vi "generateSweep.vi"(0 "Sweep type":u16(ring) items=["Linear", "Logarithmic"], 5 "Points or Points/Decade":u16=10 min=1 step=1, 7 "Start frequency":dbl=1000.0 min=0.0 step=1000.0 format="%.2p", 9 "Stop frequency":dbl=10000.0 min=0.0 step=1000.0 format="%.2p", 11 "error in (no error)":errorcluster) -> (4 "Sweep values":dbl[](array[numeric]) format="%_6g", 6 "Count":u32, 15 "error out":errorcluster)   [LabVIEW 2020]
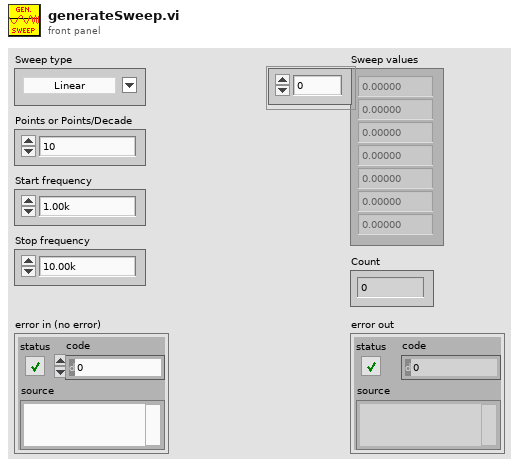
[diagram p1: front panel]
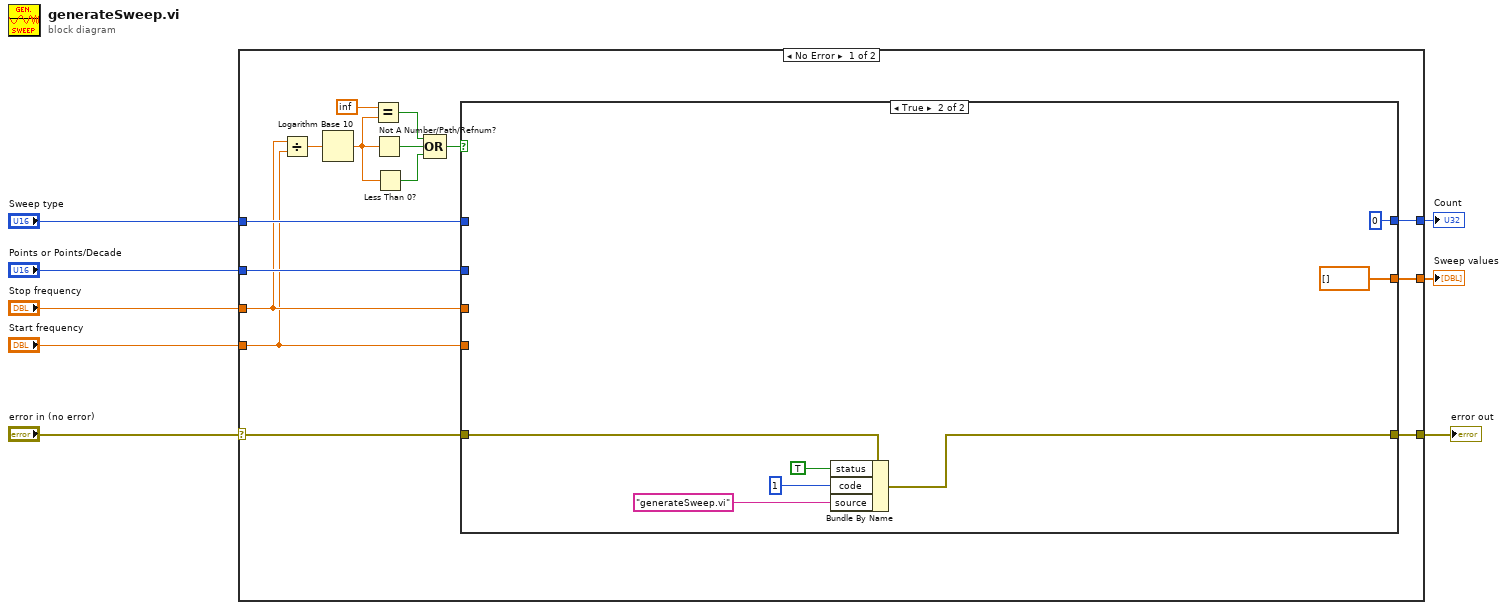
[diagram p0: block diagram]
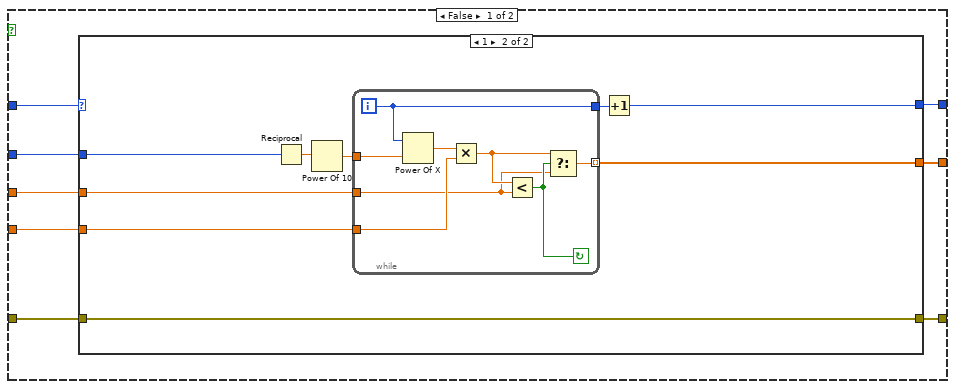
[diagram p2: hidden frame]
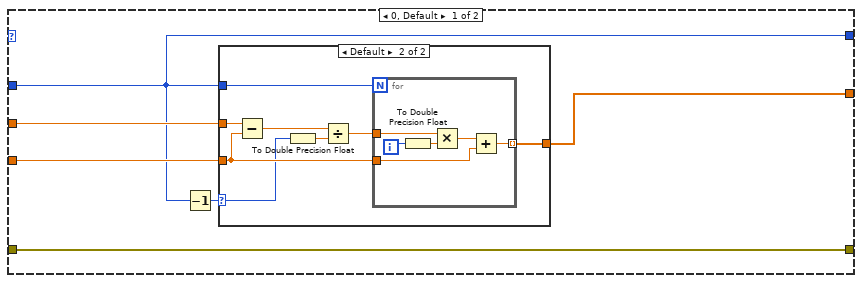
[diagram p3: hidden frame]
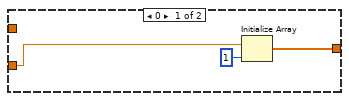
[diagram p4: hidden frame]
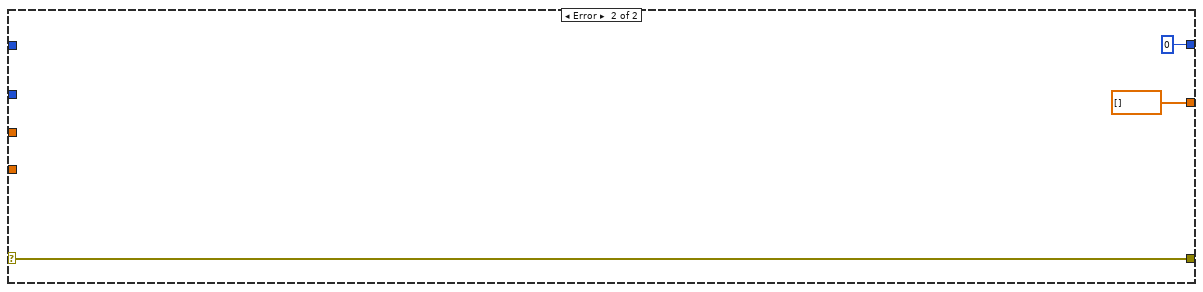
[diagram p5: hidden frame]
diagram:
  n1 = case shown="No Error" "error in (no error)" {
    selector: "error in (no error)" -> [w21 w81]
    tunnel: "Sweep type" -> [w23 _]
    tunnel: "Points or Points/Decade" -> [w22 _]
    tunnel: "Stop frequency" -> [w12 _]
    tunnel: "Start frequency" -> [w11 _]
    tunnel: [w20 w81] -> w3
    tunnel: [w10 0 ("Points or Points/Decade")] -> w2
    tunnel: [w9 dbl[] []] -> w1
    frame No Error {
      n2 = Divide(x=w12, y=w11) -> (x/y=w19:dbl)
      n3 = Logarithm Base 10(1:w19) -> (0:w14:dbl)
      n4 = Equal?(x=inf, y=w14) -> (x = y?=w18:bool)
      n5 = Not A Number/Path/Refnum?(number/path/refnum=w14) -> (NaN/Path/Refnum?=w17:bool)
      n6 = Less Than 0?(x=w14) -> (x < 0?=w16:bool)
      n7 = Compound Arithmetic op=OR(w18, w17, w16) -> (w13:bool)
      n8 = case shown="True" w13 {
        tunnel: w23 -> [w31 _]
        tunnel: w22 -> [w30 _]
        tunnel: w12 -> [w29 _]
        tunnel: w11 -> [w28 _]
        tunnel: w21 -> [w27 w75]
        tunnel: [w26 w74] -> w20
        tunnel: [w25 0 ("Points or Points/Decade")] -> w10
        tunnel: [w24 dbl[] []] -> w9
        frame False {
          n9 = case shown="1" w31 {
            tunnel: w30 -> [w32 w59]
            tunnel: w28 -> [w36 w57]
            tunnel: w29 -> [w35 w58]
            tunnel: w27 -> [w33 w63]
            tunnel: [w33 w63] -> w26
            tunnel: [w32 w56] -> w25
            tunnel: [w34 w55] -> w24
            frame 0, Default {
              n10 = Decrement(x=w32) -> (x-1=w37:u16)
              n11 = case shown="Default" w37 {
                selector: w37 -> [_ w43]
                tunnel: w35 -> [_ w48]
                tunnel: w36 -> [w38 w44]
                tunnel: [w40 w42] -> w34
                tunnel: w32 -> [_ w41]
                frame 0 {
                  n12 = Initialize Array(w38, 1 ("dimension size")) -> (w40:dbl[])
                }
                frame Default {
                  n13 = Subtract(x=w48, y=w44) -> (x-y=w47:dbl)
                  n14 = To Double Precision Float(number=w43) -> (double precision float=w46:dbl)
                  n15 = Divide(x=w47, y=w46) -> (x/y=w45:dbl)
                  n16 = for {
                    N: w41 -> [_]
                    tunnel: w45 -> [w53]
                    tunnel: w44 -> [w54]
                    tunnel: [w49] -> w42 mode=indexing
                    i -> [w52]
                    n17 = To Double Precision Float(number=w52) -> (double precision float=w50:dbl)
                    n18 = Multiply(x=w53, y=w50) -> (x*y=w51:dbl)
                    n19 = Add(x=w51, y=w54) -> (x+y=w49:dbl)
                  }
                }
              }
            }
            frame 1 {
              n20 = Reciprocal(x=w59) -> (1/x=w62:dbl)
              n21 = Power Of 10(x=w62) -> (10^x=w61:dbl)
              n22 = while {
                tunnel: w61 -> [w68]
                tunnel: w57 -> [w71]
                tunnel: [w67] -> w55 mode=indexing
                tunnel: [w69] -> w60
                tunnel: w58 -> [w64]
                i -> [w69]
                stop <- w66 continue-if-true
                n23 = Power Of X(1:w68, 2:w69) -> (0:w70:dbl)
                n24 = Multiply(x=w70, y=w71) -> (x*y=w65:dbl)
                n25 = Less?(x=w65, y=w64) -> (x < y?=w66:bool)
                n26 = Select(t=w65, s=w66, f=w64) -> (s? t:f=w67:dbl)
              }
              n27 = Increment(x=w60) -> (x+1=w56:i32)
            }
          }
        }
        frame True {
          n28 = Bundle By Name(cluster=w75, "status"=TRUE, "code"=1, "source"="generateSweep.vi") -> (w74:errorcluster)
        }
      }
    }
    frame Error {
    }
  }
  "error out" <- w3
  "Count" <- w2
  "Sweep values" <- w1
